vi "test list submodule.vi"   [LabVIEW 2017]
uses:
  user.lib/_NEVSTOP/Communicable State Machine(CSM)/Communicable State Machine.lvlib
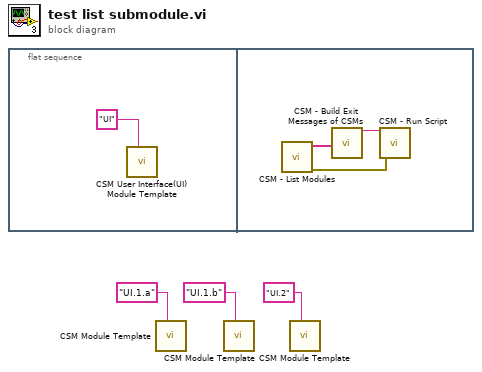
[diagram p0: block diagram]
diagram:
  n1 = flat-sequence {
    frame #0 {
      n2 = call "CSM User Interface(UI) Module Template.vi"("Name (\"\" to Use UUID)"="UI" ("Name(\"\" to use uuid)")) -> ()  [unwired: 11 in]
    }
    frame #1 {
      n3 = call "CSM - List Modules.vi"() -> ("error out"=w5:errorcluster, "Module Names"=w7:string[])  [unwired: 10 in]
      n4 = call "CSM - Build Exit Messages of CSMs.vi"("CSMs"=w7) -> ("States"=w6:string)  [unwired: 14 in]
      n5 = call "CSM - Run Script.vi"("CSM Scripts"=w6, "error in (no error)"=w5) -> ()  [unwired: 11 in, 3 out]
    }
  }
  n6 = call "CSM Module Template.vi"("Name (\"\" to Use UUID)"="UI.1.a" ("Name(\"\" to use uuid)")) -> ()  [unwired: 11 in]
  n7 = call "CSM Module Template.vi"("Name (\"\" to Use UUID)"="UI.1.b" ("Name(\"\" to use uuid)")) -> ()  [unwired: 11 in]
  n8 = call "CSM Module Template.vi"("Name (\"\" to Use UUID)"="UI.2" ("Name(\"\" to use uuid)")) -> ()  [unwired: 11 in]
